vi "RichToFlatstreamtest_StreamData.vi"(5 "OutputClusterType":T1, 11 "InputCluster":T2) -> (3 "OutputCluster":T1)   [LabVIEW 2021, in "streamtest_server.lvlib"]
uses:
  streamtest_server.lvlib
  streamtest_StreamData.ctl
  streamtest_StreamData_Flat.ctl
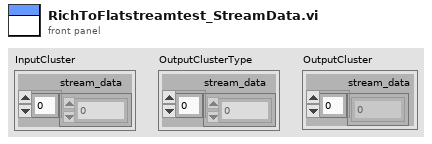
[diagram p1: front panel]
types:
  T1 = typedef "streamtest_server.lvlib/streamtest_StreamData_Flat.ctl" = cluster{"stream_data":u8[]}
  T2 = typedef "streamtest_server.lvlib/streamtest_StreamData.ctl" = cluster{"stream_data":u8[]}
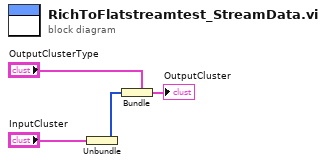
[diagram p0: block diagram]
diagram:
  n1 = Unbundle "Unbundle"("InputCluster") -> ("stream_data"=w1:u8[])
  n2 = Bundle "Bundle"(cluster="OutputClusterType", "stream_data"=w1) -> (→"OutputCluster":T1)
